vi "Get JPG RGB Channel(Demo).vi"() -> ()   [LabVIEW 2012, in "Picture Box Tools.lvlib"]
uses:
  Picture Box Tools.lvlib
panel:
  out "Origin Picture":picture caption="源图片"
  out "Channel picture":picture caption="通道图片"
  in  "模式":enum16{"Red", "Green", "Blue"}(ring)
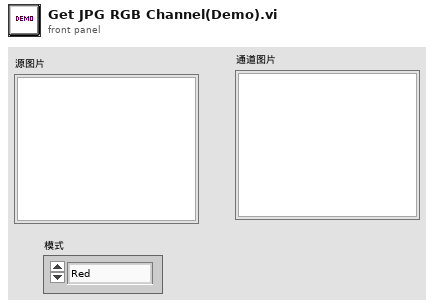
[diagram p1: front panel]
types:
  T1 = typedef "imagedata.ctl" = cluster{"image type":i32, "image depth":i32, "image":u8[], "mask":u8[], "colors":u32[], "Rectangle":cluster{"left":i16, "top":i16, "right":i16, "bottom":i16}}
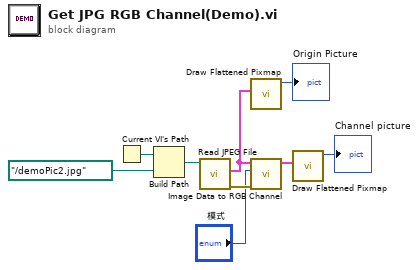
[diagram p0: block diagram]
diagram:
  n1 = Current VI's Path() -> (path=w9:path)
  n2 = Build Path(base path=w9, name or relative path=path "../demoPic2.jpg") -> (appended path=w7:path)
  n3 = call <vilib>:"Read JPEG File.vi"("path to JPEG file"=w7) -> ("error out"=w6:errorcluster, "image data"=w2:T1)  [unwired: 8 in, 1 out]
  n4 = call <vilib>:"Draw Flattened Pixmap.vi"("image data"=w2) -> ("new picture"=→"Origin Picture":picture)  [unwired: 8 in]
  n5 = call "Image Data to RGB Channel.vi"("错误输入"=w6, "模式"="模式", "image data In"=w2) -> ("image data Out"=w4:T1)  [unwired: 7 in, 1 out]
  n6 = call <vilib>:"Draw Flattened Pixmap.vi"("image data"=w4) -> ("new picture"=→"Channel picture":picture)  [unwired: 8 in]
